vi "UDPrecieverLoop.vi"() -> ()   [LabVIEW 2012]
panel:
  out "Array":bool[][](array[boolean])
  out "size(s)":i32
  out "number":u32
  out "data pre process":u32
  out "packet in \nconstruction":u32
  out "data process":u32
  out "packet constructed":u32
  out "packet\nprocess":u32
  out "UDP reciever\nloop":u32
  out "start time":u32
  out "channel 11":u32[](graph)
  out "in 11":bool
  out "channel 10":u32[](graph)
  out "in 10":bool
  out "channel 9":u32[](graph)
  out "in 9":bool
  out "channel 8":u32[](graph)
  out "in 8":bool
  out "channel 7":u32[](graph)
  out "in 7":bool
  out "channel 6":u32[](graph)
  out "in 6":bool
  out "channel 5":u32[](graph)
  out "in 5":bool
  out "channel 4":u32[](graph)
  out "in 4":bool
  out "channel 3":u32[](graph)
  out "in 3":bool
  out "channel 2":u32[](graph)
  out "in 2":bool
  out "channel 1":u32[](graph)
  out "in 1":bool
  out "channel 0":u32[](graph)
  out "in 0":bool
  out "NumBins":u32
  out "Cnts/Bin":u32
  out "Prof/Hist":u32
  out "Sync":u32
  out "Channel":u32
  out "rTime":u32
  out "frameCntr":u32
  out "built packet array":string[](array[string])
  out "channel":u32
  out "Found Header":bool
  out "Raw Data Out":string
  out "error post-check":errorcluster
  out "End Reciever Error":errorcluster
  in  "stop reciever":bool
  out "port":u16
  out "error out post-read":errorcluster
  out "error out pre-read":errorcluster
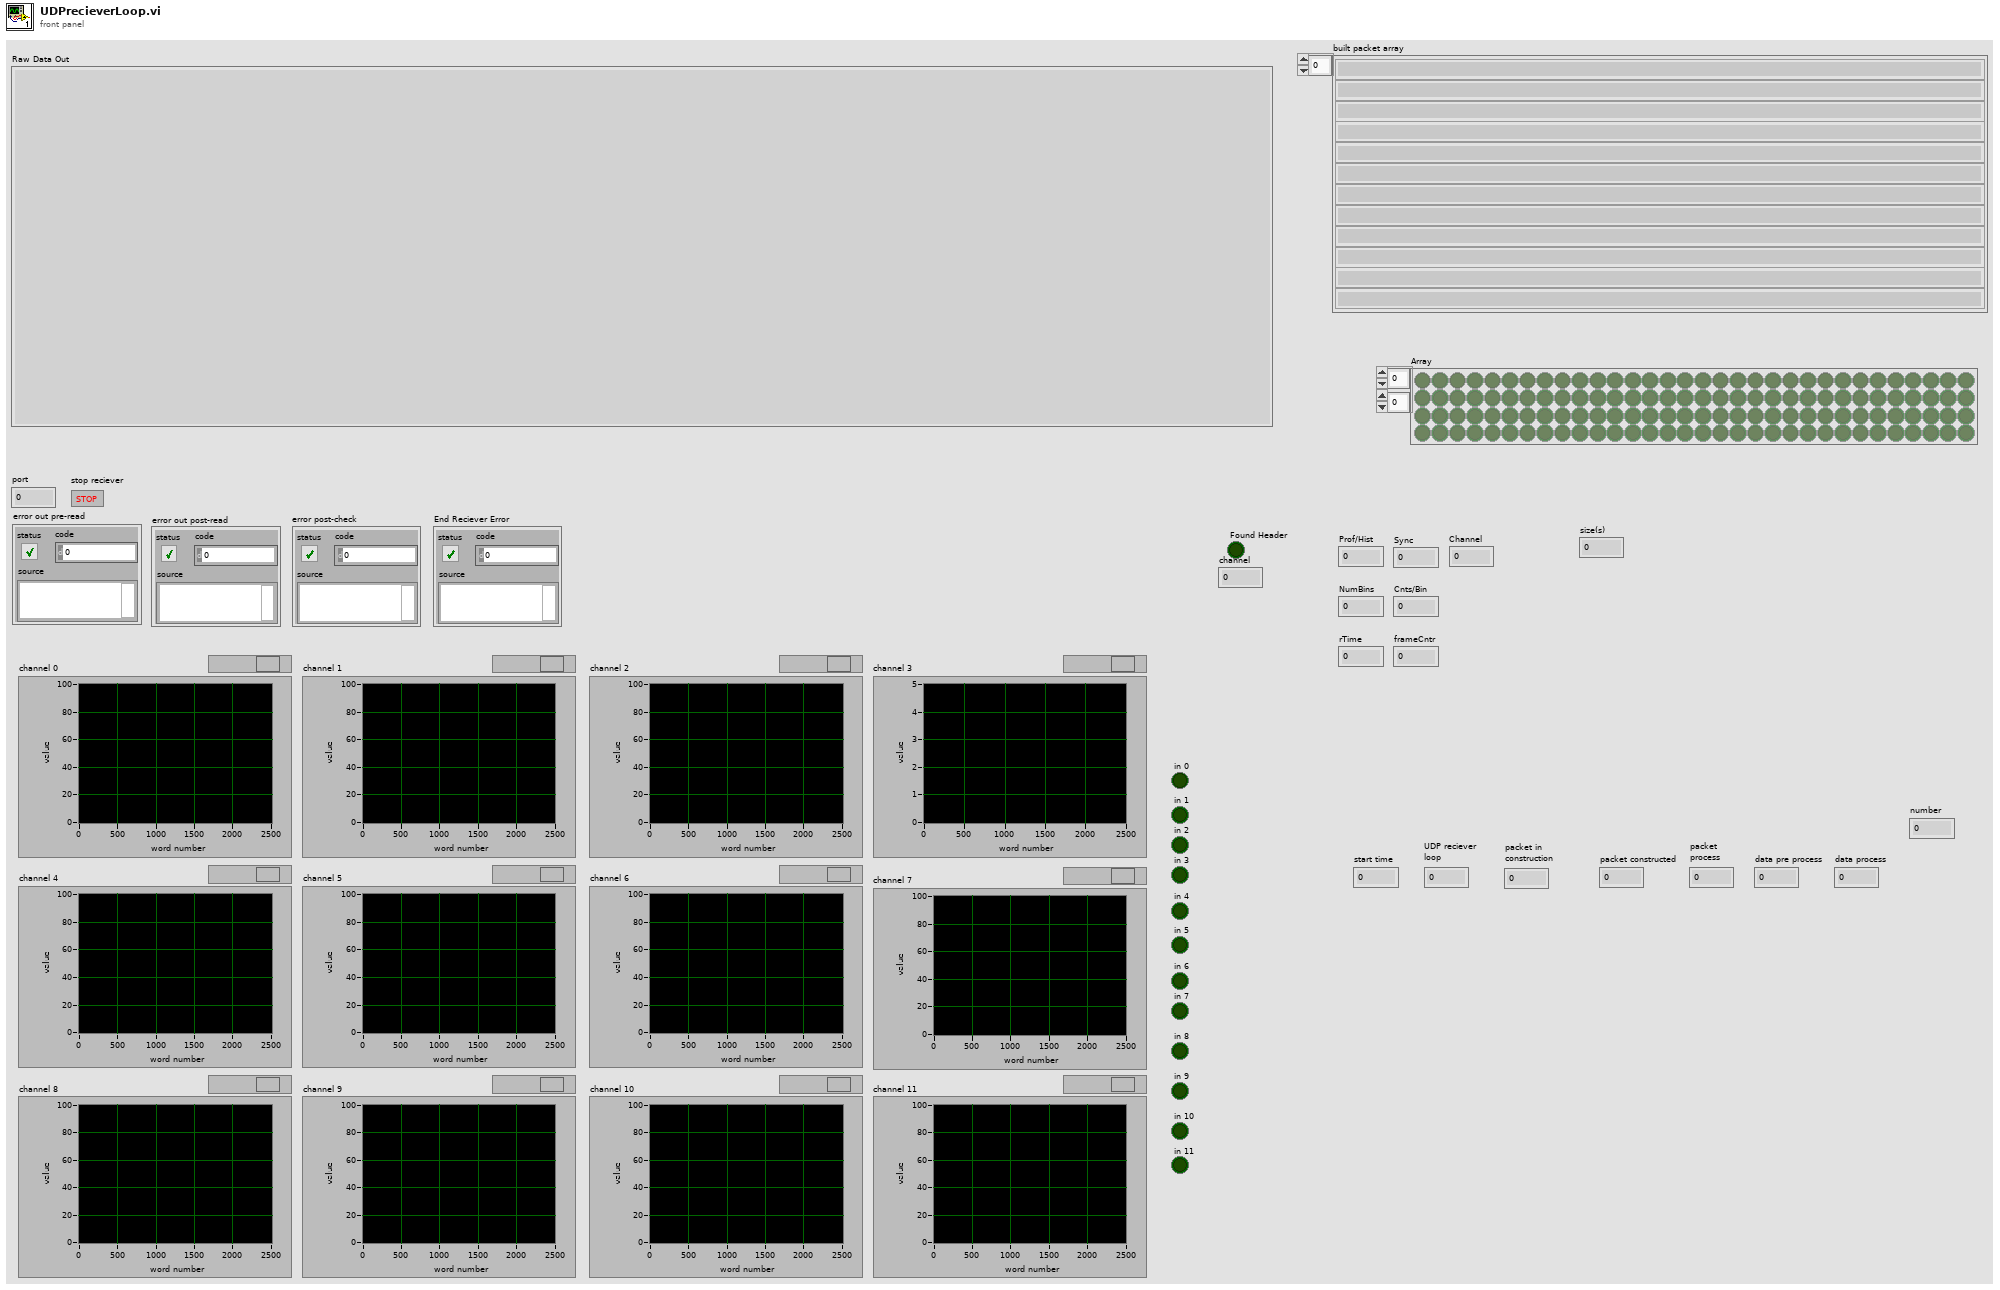
[diagram p1: front panel]
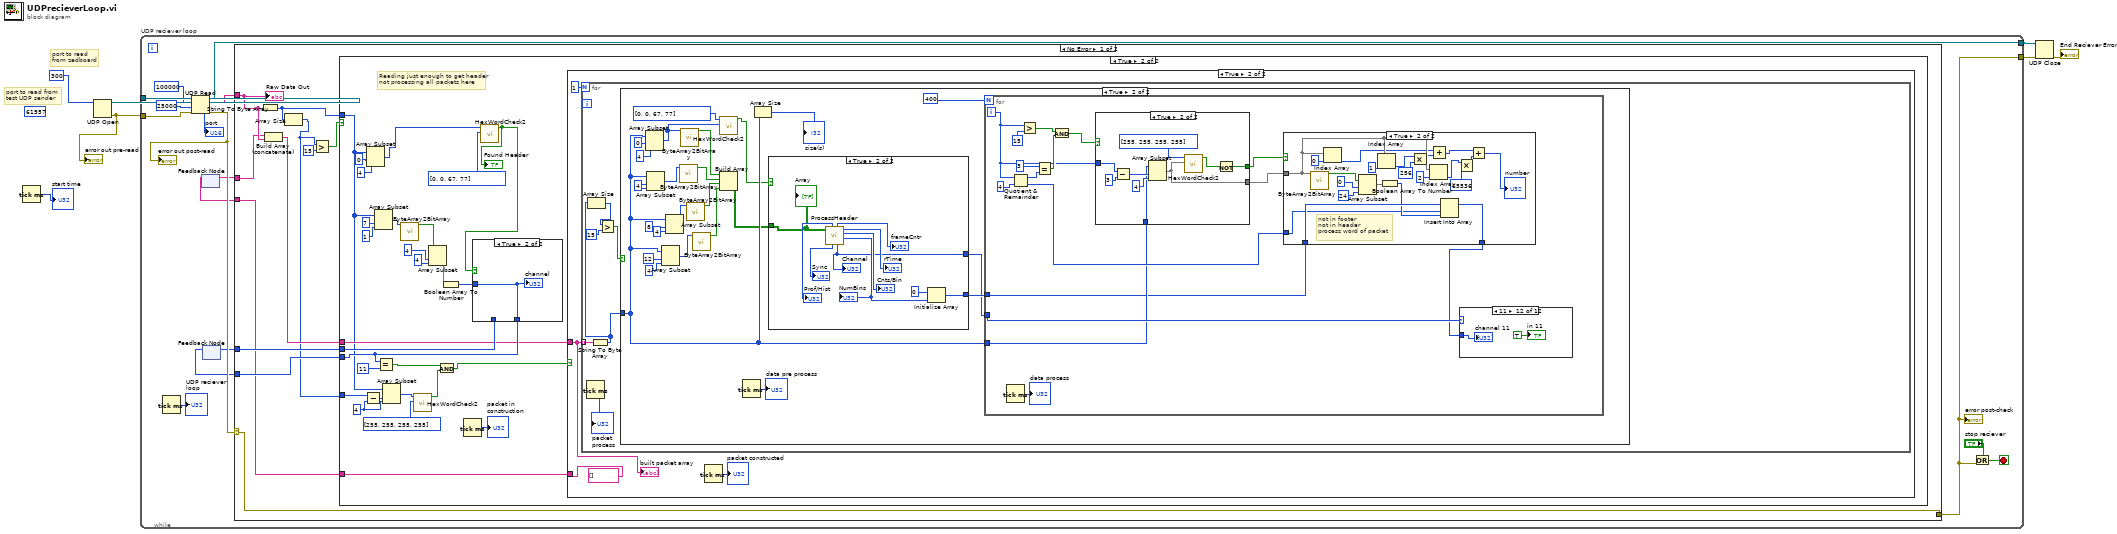
[diagram p0: block diagram]
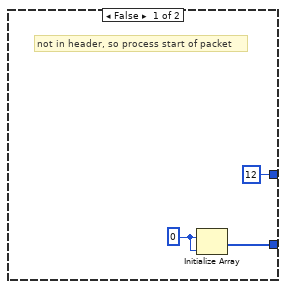
[diagram p5: hidden frame]
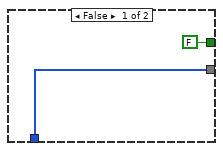
[diagram p6: hidden frame]
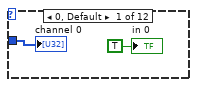
[diagram p7: hidden frame]
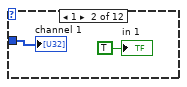
[diagram p8: hidden frame]
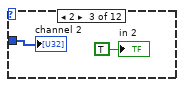
[diagram p9: hidden frame]
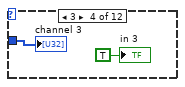
[diagram p10: hidden frame]
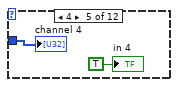
[diagram p11: hidden frame]
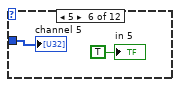
[diagram p12: hidden frame]
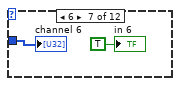
[diagram p13: hidden frame]
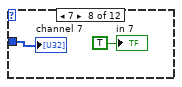
[diagram p14: hidden frame]
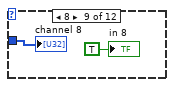
[diagram p15: hidden frame]
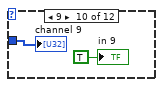
[diagram p16: hidden frame]
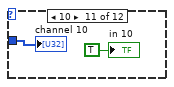
[diagram p17: hidden frame]
diagram:
  (unwired) u16 61557 ("port")
  # "port to read \nfrom zedboard"
  # "port to read from \ntest UDP sender"
  n1 = Tick Count (ms)() -> (millisecond timer value=→"start time":u32)
  n2 = UDP Open(11:u16 300 ("port")) -> (port=w6:refnum<k16>, 0:w3:errorcluster)  [unwired: 4 in, 1 out]
  "error out pre-read" <- w3
  n3 = while "UDP reciever loop" {
    tunnel: [w23] -> w7
    tunnel: w6 -> [w22]
    tunnel: [w14] -> w5
    tunnel: w3 -> [w19]
    stop <- w21 stop-if-true
    n4 = Tick Count (ms)() -> (millisecond timer value=→"UDP reciever\nloop":u32)
    n5 = UDP Read(connection ID=w22, max size (548)=100000, timeout ms (25000)=25000, 8:w19) -> (data out=w16:string, error out=w18:errorcluster, 3:w23:refnum<k16>, 4:→"port":u16)  [unwired: 1 out]
    "error out post-read" <- w18
    n6 = feedback #1() -> (w11:string[])  [unwired: 1 in]
    n7 = feedback #2() -> (w9:u32)  [unwired: 1 in]
    n8 = case shown="No Error" w18 {
      selector: w18 -> [w34 w190]
      tunnel: w16 -> [w33 _]
      tunnel: [w34 w190] -> w14
      tunnel: [w25 w189] -> w12
      tunnel: w11 -> [w32 w189]
      tunnel: [w29 w188] -> w10
      tunnel: w9 -> [w28 w188]
      frame No Error {
        n9 = String To Byte Array(string=w33) -> (unsigned byte array=w26:u8[])
        n10 = Build Array (concatenate)(w32, w33) -> (w27:string[])
        n11 = Array Size(array=w26) -> (size(s)=w24:i32)
        n12 = Greater?(x=w24, y=15) -> (0:w31:bool)
        n13 = case shown="True" w31 {
          tunnel: w26 -> [_ w46]
          tunnel: [w36 w50] -> w29
          tunnel: w28 -> [w36 w51]
          tunnel: w24 -> [_ w54]
          tunnel: w27 -> [w35 w48]
          tunnel: [w35 w47] -> w25
          frame False {
          }
          frame True {
            w56 = 4 ("length")
            # "Reading just enough to get header\nnot processing all packets here"
            n14 = Subtract(x=w54, y=w56) -> (x-y=w55:i32)
            n15 = Array Subset(array=w46, index=0, length=4) -> (w60:u8[])
            n16 = Array Subset(array=w46, index=7, length=1) -> (w43:u8[])
            n17 = Array Subset(array=w46, index=w55, length=w56) -> (w49:u8[])
            n18 = call "ByteArray2BitArray.vi"("array"=w43) -> ("Array"=w40:bool[])  [unwired: 10 in]
            n19 = call "HexWordCheck2.vi"("array"=u8[] [255, 255, 255, 255], "Input Array"=w49) -> ("Boolean"=w57:bool)  [unwired: 9 in]
            n20 = Array Subset(array=w40, index=4, length=4) -> (w38:bool[])
            n21 = Boolean Array To Number(Boolean array=w38) -> (number=w39:u32)
            n22 = Tick Count (ms)() -> (millisecond timer value=→"packet in \nconstruction":u32)
            n23 = call "HexWordCheck2.vi"("array"=u8[] [0, 0, 67, 77], "Input Array"=w60) -> ("Boolean"=w61:bool)  [unwired: 9 in]
            "Found Header" <- w61
            n24 = case shown="True" w61 {
              tunnel: [w186 w187] -> w50
              tunnel: w51 -> [w186 _]
              tunnel: w39 -> [_ w187]
              frame False {
              }
              frame True {
                "channel" <- w187
              }
            }
            n25 = Equal?(x=w50, y=u32 11) -> (x = y?=w53:bool)
            n26 = And(x=w53, y=w57) -> (x .and. y?=w58:bool)
            n27 = case shown="True" w58 {
              tunnel: w48 -> [w65 w68]
              tunnel: [w65 string[] []] -> w47
              frame False {
              }
              frame True {
                n28 = for {
                  N: 1 -> [_]
                  tunnel: w68 -> [w75] mode=indexing
                  n29 = Tick Count (ms)() -> (millisecond timer value=→"packet\nprocess":u32)
                  n30 = String To Byte Array(string=w75) -> (unsigned byte array=w74:u8[])
                  n31 = Array Size(array=w74) -> (size(s)=w73:i32)
                  n32 = Greater?(x=w73, y=15) -> (0:w71:bool)
                  n33 = case shown="True" w71 {
                    tunnel: w74 -> [_ w83]
                    frame False {
                    }
                    frame True {
                      w88 = 4 ("length")
                      n34 = Array Subset(array=w83, index=0, length=4) -> (w98:u8[])
                      n35 = Array Subset(array=w83, index=w88, length=w88) -> (w84:u8[])
                      n36 = Array Subset(array=w83, index=12, length=4) -> (w97:u8[])
                      n37 = Array Subset(array=w83, index=8, length=4) -> (w85:u8[])
                      n38 = call "ByteArray2BitArray.vi"("array"=w84) -> ("Array"=w94:bool[])  [unwired: 10 in]
                      n39 = call "ByteArray2BitArray.vi"("array"=w98) -> ("Array"=w93:bool[])  [unwired: 10 in]
                      n40 = call "ByteArray2BitArray.vi"("array"=w85) -> ("Array"=w96:bool[])  [unwired: 10 in]
                      n41 = call "ByteArray2BitArray.vi"("array"=w97) -> ("Array"=w95:bool[])  [unwired: 10 in]
                      n42 = call "HexWordCheck2.vi"("array"=w98, "Input Array"=u8[] [0, 0, 67, 77] ("array")) -> ("Boolean"=w82:bool)  [unwired: 9 in]
                      n43 = Build Array(w93, w94, w96, w95) -> (w81:bool[][])
                      n44 = Tick Count (ms)() -> (millisecond timer value=→"data pre process":u32)
                      n45 = Array Size(array=w83) -> (size(s)=→"size(s)":i32)
                      n46 = case shown="True" w82 {
                        tunnel: w81 -> [_ w106]
                        tunnel: [w102 w105] -> w80
                        tunnel: [u32 12 ("Numeric 4") w103] -> w79
                        frame False {
                          w100 = u32 0 ("element")
                          # "not in header, so process start of packet"
                          n47 = Initialize Array(w100, w100) -> (w102:u32[])
                        }
                        frame True {
                          n48 = call "ProcessHeader.vi"("Array"=w106) -> ("Numeric"=w107:u32, "Numeric 7"=→"Cnts/Bin":u32, "Numeric 3"=→"rTime":u32, "Numeric 4"=w103:u32, "Numeric 2"=→"frameCntr":u32, "Numeric 5"=→"Sync":u32, "Numeric 6"=→"Prof/Hist":u32)  [unwired: 4 in]
                          "NumBins" <- w107
                          "Channel" <- w103
                          n49 = Initialize Array(u32 0 ("element"), w107) -> (w105:u32[])
                          "Array" <- w106
                        }
                      }
                      n50 = for {
                        N: 400 -> [_]
                        tunnel: w83 -> [w116]
                        tunnel: w80 -> [w115]
                        tunnel: w79 -> [w126]
                        i -> [w113]
                        n51 = Tick Count (ms)() -> (millisecond timer value=→"data process":u32)
                        n52 = Quotient & Remainder(x=w113, y=4) -> (x-y*floor(x/y)=w122:i32, floor(x/y)=w124:i32)
                        n53 = Greater?(x=w113, y=15 ("x")) -> (0:w121:bool)
                        n54 = Equal?(x=3, y=w122) -> (x = y?=w120:bool)
                        n55 = And(x=w121, y=w120) -> (x .and. y?=w119:bool)
                        n56 = case shown="True" w119 {
                          tunnel: w116 -> [w129 w135]
                          tunnel: [FALSE ("Boolean") w132] -> w117
                          tunnel: [w129 w134] -> w118
                          tunnel: w113 -> [_ w133]
                          frame False {
                          }
                          frame True {
                            n57 = Subtract(x=w133, y=3) -> (x-y=w138:i32)
                            n58 = Array Subset(array=w135, index=w138, length=4) -> (w134:u8[])
                            n59 = call "HexWordCheck2.vi"("array"=w134, "Input Array"=u8[] [255, 255, 255, 255] ("array")) -> ("Boolean"=w131:bool)  [unwired: 9 in]
                            n60 = Not(x=w131) -> (.not. x?=w132:bool)
                          }
                        }
                        n61 = case shown="True" w117 {
                          tunnel: w115 -> [w164 w185]
                          tunnel: w118 -> [_ w174]
                          tunnel: [w164 w179] -> w125
                          tunnel: w124 -> [_ w178]
                          frame False {
                          }
                          frame True {
                            # "not in footer \nnot in header\nprocess word of packet"
                            n62 = call "ByteArray2BitArray.vi"("array"=w174) -> ("Array"=w180:bool[])  [unwired: 10 in]
                            n63 = Index Array(array=w174, index=0) -> (element=w173:u8)
                            n64 = Array Subset(array=w180, index=0, length=24) -> (w182:bool[])
                            n65 = Index Array(array=w174, index=1) -> (element=w171:u8)
                            n66 = Boolean Array To Number(Boolean array=w182) -> (number=w181:u32)
                            n67 = Multiply(x=w171, y=256) -> (x*y=w172:i32)
                            n68 = Index Array(array=w174, index=2) -> (element=w167:u8)
                            n69 = Add(x=w173, y=w172) -> (x+y=w169:i32)
                            n70 = Insert Into Array(array=w185, index=w178, new element=w181) -> (w179:u32[])
                            n71 = Multiply(x=w167, y=65536) -> (x*y=w168:i32)
                            n72 = Add(x=w169, y=w168) -> (x+y=→"number":i32)
                          }
                        }
                        n73 = case shown="11" w126 {
                          tunnel: w125 -> [w141 w143 w145 w147 w149 w151 w153 w155 w157 w159 w161 w163]
                          frame 0, Default {
                            "channel 0" <- w141
                            "in 0" <- TRUE ("in 11")
                          }
                          frame 1 {
                            "channel 1" <- w143
                            "in 1" <- TRUE ("in 11")
                          }
                          frame 2 {
                            "channel 2" <- w145
                            "in 2" <- TRUE ("in 11")
                          }
                          frame 3 {
                            "channel 3" <- w147
                            "in 3" <- TRUE ("in 11")
                          }
                          frame 4 {
                            "channel 4" <- w149
                            "in 4" <- TRUE ("in 11")
                          }
                          frame 5 {
                            "channel 5" <- w151
                            "in 5" <- TRUE ("in 11")
                          }
                          frame 6 {
                            "channel 6" <- w153
                            "in 6" <- TRUE ("in 11")
                          }
                          frame 7 {
                            "channel 7" <- w155
                            "in 7" <- TRUE ("in 11")
                          }
                          frame 8 {
                            "channel 8" <- w157
                            "in 8" <- TRUE ("in 11")
                          }
                          frame 9 {
                            "channel 9" <- w159
                            "in 9" <- TRUE ("in 11")
                          }
                          frame 10 {
                            "channel 10" <- w161
                            "in 10" <- TRUE ("in 11")
                          }
                          frame 11 {
                            "channel 11" <- w163
                            "in 11" <- TRUE ("in 11")
                          }
                        }
                      }
                    }
                  }
                }
                n74 = Tick Count (ms)() -> (millisecond timer value=→"packet constructed":u32)
                "built packet array" <- w68
              }
            }
          }
        }
        "Raw Data Out" <- w33
      }
      frame Error {
      }
    }
    "error post-check" <- w14
    n75 = feedback-in #1(w12) -> ()
    n76 = feedback-in #2(w10) -> ()
    n77 = Or(x="stop reciever", y=w14) -> (x .or. y?=w21:bool)
  }
  n78 = UDP Close(connection ID=w7, 8:w5) -> (error out=→"End Reciever Error":errorcluster)  [unwired: 1 out]
